vi "AppleScript Main.vi"   [LabVIEW 2016, in "Apple script.lvlib"]
doc: "Main block for AppleScript.\nPut this in the autonomous vi. Do not place this inside of a loop."
uses:
  Apple script.lvlib
  <vilib>/Rock Robotics/Network Tables/NT Read String.vi
  <vilib>/Rock Robotics/Network Tables/NT Read Number.vi
panel:
  # "AppleScript\nAutonomous Scripting Language for LabVIEW\nCreated by Cory Lynch\nFRC Team 2067"
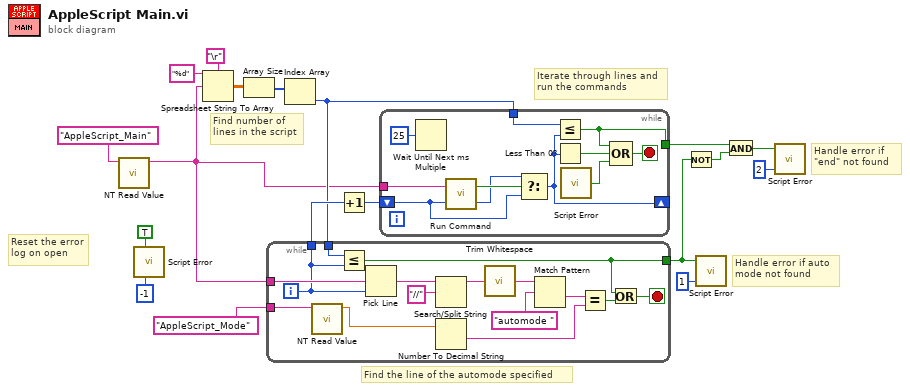
[diagram p0: block diagram]
diagram:
  # "Find number of \nlines in the script"
  # "Handle error if\n\"end\" not found"
  # "Handle error if auto\nmode not found"
  # "Iterate through lines and\nrun the commands"
  # "Find the line of the automode specified"
  # "Reset the error\nlog on open"
  n1 = call-poly <vilib>:"NT Read Value.vi"("Name"="AppleScript_Main") -> ("String"=w2:string)  [unwired: 9 in, 1 out]
  n2 = call "Script Error.vi"("Reset Log"=TRUE, "Line Number"=-1) -> ()  [unwired: 3 in, 1 out]
  n3 = Spreadsheet String To Array(delimiter (Tab)="\r", format string="%d", spreadsheet string=w2) -> (array=w17:dbl[][])  [unwired: 1 in]
  n4 = Array Size(array=w17) -> (size(s)=w14:i32[])
  n5 = Index Array(array=w14) -> (element=w8:i32)  [unwired: 1 in]
  n6 = while {
    tunnel: w2 -> [w27]
    tunnel: [w23] -> w18
    tunnel: w8 -> [w24]
    tunnel: [w21] -> w7
    tunnel: "AppleScript_Mode" ("Name") -> [w19]
    i -> [w23]
    stop <- w22 stop-if-true
    n7 = call-poly <vilib>:"NT Read Value.vi"("Name"=w19) -> ("Numeric"=w20:dbl)  [unwired: 9 in, 1 out]
    n8 = Less Or Equal?(x=w24, y=w23) -> (x <= y?=w21:bool)
    n9 = Pick Line(multi-line string=w27, line index=w23) -> (output string=w26:string)  [unwired: 1 in]
    n10 = Search/Split String(string=w26, search string/char (-)="//") -> (substring before match=w29:string)  [unwired: 1 in, 2 out]
    n11 = Number To Decimal String(number=w20) -> (decimal integer string=w31:string)  [unwired: 1 in]
    n12 = call <vilib>:"Trim Whitespace.vi"("string"=w29) -> ("trimmed string"=w28:string)  [unwired: 1 in]
    n13 = Match Pattern(string=w28, regular expression="automode ") -> (after substring=w32:string)  [unwired: 1 in, 3 out]
    n14 = Equal?(x=w32, y=w31) -> (x = y?=w25:bool)
    n15 = Or(x=w21, y=w25) -> (x .or. y?=w22:bool)
  }
  n16 = Increment(x=w18) -> (x+1=w5:i32)
  n17 = while {
    tunnel: w2 -> [w44]
    shift-right: [w41] -> _
    shift-left: w5 -> [w43]
    tunnel: w8 -> [w40]
    tunnel: [w39] -> w11
    stop <- w37 stop-if-true
    n18 = Wait Until Next ms Multiple(millisecond multiple=u32 25 ("milliseconds to wait")) -> ()  [unwired: 1 out]
    n19 = call "Run Command.vi"("Line Index In"=w43, "Script"=w44) -> ("Line Index Out"=w34:i32, "Done"=w42:bool)
    n20 = Select(t=w34, s=w42, f=w43) -> (s? t:f=w41:i32)
    n21 = Less Or Equal?(x=w40, y=w41) -> (x <= y?=w39:bool)
    n22 = Less Than 0?(x=w41) -> (x < 0?=w38:bool)
    n23 = call "Script Error.vi"() -> ("Error?"=w36:bool)  [unwired: 5 in]
    n24 = Compound Arithmetic op=OR(w39, w38, w36) -> (w37:bool)
  }
  n25 = Not(x=w7) -> (.not. x?=w10:bool)
  n26 = call "Script Error.vi"("Error?"=w7, "Error Code"=1) -> ()  [unwired: 3 in, 1 out]
  n27 = And(x=w11, y=w10) -> (x .and. y?=w9:bool)
  n28 = call "Script Error.vi"("Error?"=w9, "Error Code"=2) -> ()  [unwired: 3 in, 1 out]
